vi "TTA_MATLAB_RFIC_SetDGAttTest_DetailedResults.vi"(7 "Tx Result":cluster{"TX1":dbl[], "TXx3":dbl[]}[](array[cluster]), 8 "error in":errorcluster, 10 "TestGroup":string, 11 "SubTest":string) -> (0 "error out":errorcluster, 3 "SubTestSuccess":dbl[](array[numeric]))   [LabVIEW 2016]
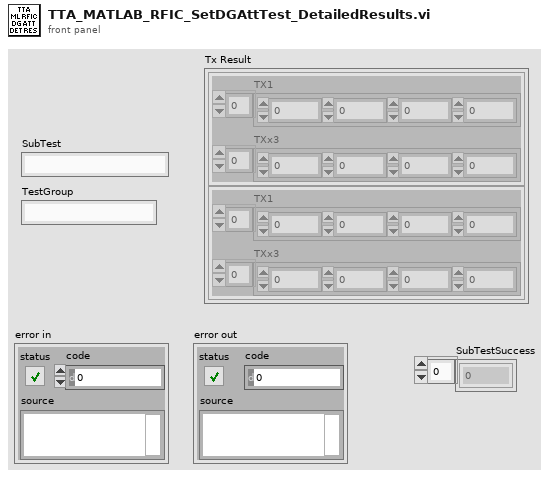
[diagram p1: front panel]
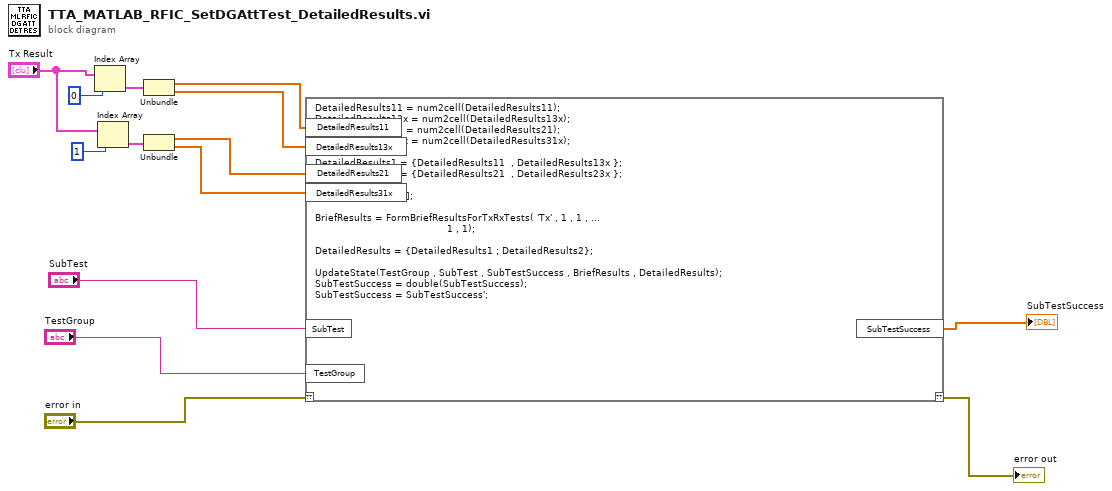
[diagram p0: block diagram]
diagram:
  n1 = Index Array(array="Tx Result", index=0) -> (element=w6:cluster{"TX1":dbl[], "TXx3":dbl[]})
  n2 = Index Array(array="Tx Result", index=1) -> (element=w5:cluster{"TX1":dbl[], "TXx3":dbl[]})
  n3 = Unbundle(w6) -> ("TX1"=w4:dbl[], "TXx3"=w3:dbl[])
  n4 = Unbundle(w5) -> ("TX1"=w2:dbl[], "TXx3"=w1:dbl[])
  n5 = script code="DetailedResults11 = num2cell(DetailedResults11);\nDetailedResults13x = num2cell(DetailedResults13x);\nDetailedResults21 = num2cell(DetailedResults21);\nDetailedResults31x = num2cell(DetailedResults31x);\n\nDetailedResults1 = {DetailedResults11  , DetailedResults13x };\nDetailedResults2 = {DetailedResults21  , DetailedResults23x };\n\nSuccessList = [1 ;1];\n\nBriefResults = FormBriefResultsForTxRxTests( 'Tx' , 1 , 1 , ...\n                                            1 , 1);\n\nDetailedResults = {DetailedResults1 ; DetailedResults2};\n\nUpdateState(TestGroup , SubTest , SubTestSuccess , BriefResults , DetailedResults);\nSubTestSuccess = double(SubTestSuccess);\nSubTestSuccess = SubTestSuccess';"("??"="error in", "SubTest"="SubTest", "TestGroup"="TestGroup", "DetailedResults11"=w4, "DetailedResults13x"=w3, "DetailedResults21"=w2, "DetailedResults31x"=w1) -> ("??"=→"error out":errorcluster, "SubTestSuccess"=→"SubTestSuccess":dbl[])
